vi "Log Error.vi"(8 "error in (no error)":errorcluster, 10 "Error Message Data":T1, 11 "Text Log In":refnum<class "XML Log.lvclass">) -> (0 "error out":errorcluster, 3 "Text Log Out":refnum<class "XML Log.lvclass">)   [LabVIEW 2020, in "Error Log Classes.lvlib" / "XML Log.lvclass"]
uses:
  XML Log.lvclass
  Process Classes/Error Handler/Community/TypeDefs/Error Message Data.ctl
  Process Classes/Error Handler/Error Handler.lvclass
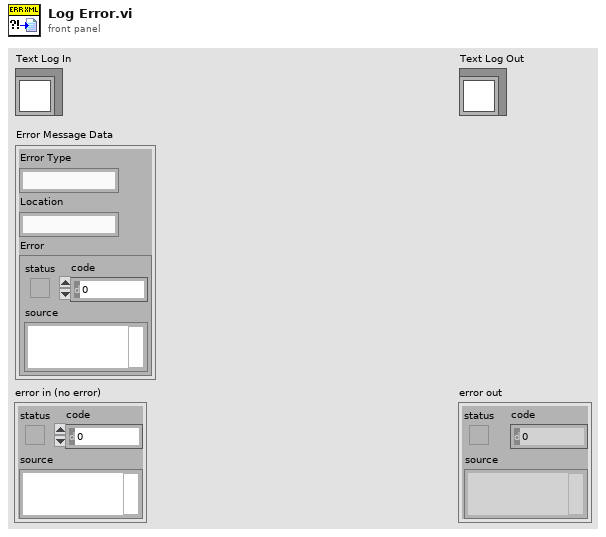
[diagram p1: front panel]
types:
  T1 = typedef "Error Handler.lvclass/Error Message Data.ctl" = cluster{"Error Type":string, "Location":string, "Error":errorcluster}
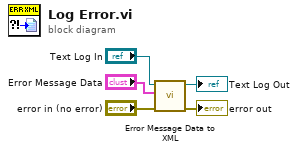
[diagram p0: block diagram]
diagram:
  n1 = call "Error Message Data to XML.vi"("error in (no error)"="error in (no error)", "Error Message Data"="Error Message Data", "Error Handler in"="Text Log In") -> ("error out"=→"error out":errorcluster, "Error Handler out"=→"Text Log Out":refnum<class "XML Log.lvclass">)  [unwired: 7 in]
